vi "setSerializedData.vi"(0 "reference":refnum<class "NoteNode.lvclass">, 1 "parent":refnum<class "AbstractNode.lvclass">, 2 "children":refnum<class "AbstractNode.lvclass">[](array[class]), 3 "xmlOut":string, 5 "error in (no error)":errorcluster) -> (14 "reference out":refnum<class "NoteNode.lvclass">, 19 "error out":errorcluster)   [LabVIEW 2020, in "NoteNode.lvclass"]
doc: "setSerializedData"
uses:
  <resource>/Framework/Providers/Open_GDS/UML/NoteNode_class/NoteNode.lvclass
  C:/Program Files (x86)/National Instruments/LabVIEW 2020/resource/Framework/Providers/Open_GDS/UML/RectangularNode_class/RectangularNode.lvclass
  C:/Program Files (x86)/National Instruments/LabVIEW 2020/resource/Framework/Providers/Open_GDS/UML/AbstractNode_class/AbstractNode.lvclass
  <resource>/Framework/Providers/Open_GDS/UML/AbstractNode_class/AbstractNode.lvclass
  <resource>/Framework/Providers/Open_GDS/UML/General/Rectangle/Rectangle Rectangle2D.ctl
  <resource>/Framework/Providers/Open_GDS/UML/MultiLineString_class/JustificationType.ctl
  <resource>/Framework/Providers/Open_GDS/UML/MultiLineString_class/MultiLineString.lvclass
  <resource>/Framework/Providers/Open_GDS/UML/RectangularNode_class/RectangularNode.lvclass
panel:
  in  "emptyPointNodes":refnum<class "AbstractNode.lvclass">[](array[class])
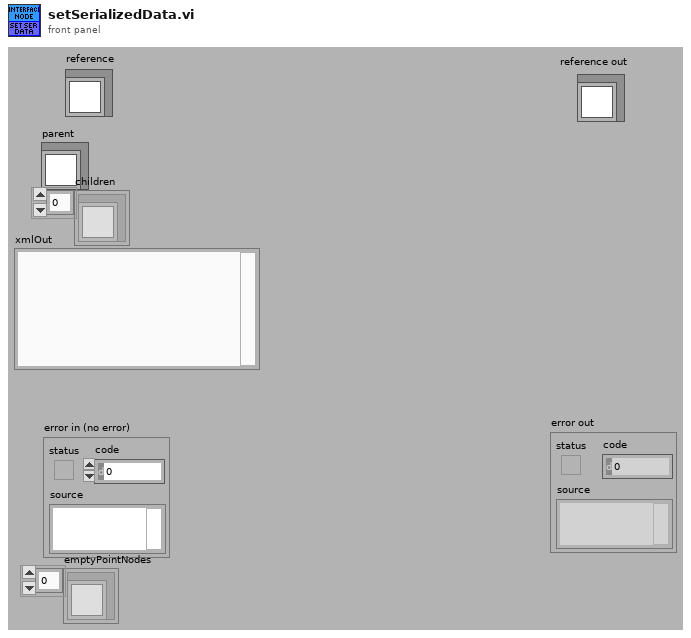
[diagram p1: front panel]
types:
  T1 = typedef "Rectangle Rectangle2D.ctl" = cluster{"x":dbl, "y":dbl, "width":dbl, "height":dbl}
  T2 = cluster{"Base class":cluster{"Base class":cluster{"parent":refnum<k1>, "children":refnum<k1>[], "Hidden":bool}, "bounds":T1}, "DEFAULT_WIDTH":i32, "DEFAULT_HEIGHT":i32, "DEFAULT_COLOR":u32, "FOLD_X":i32, "FOLD_Y":i32, "color":u32, "text":refnum<k1>, "pointNodes":refnum<k1>[]}
  T3 = typedef "MultiLineString.lvclass/JustificationType.ctl" = enum16{"LEFT", "CENTER", "RIGHT"}
  T4 = cluster{"Attributes":cluster{"Base class":cluster{"Base class":cluster{"parent":refnum<k1>, "children":refnum<k1>[], "Hidden":bool}, "bounds":T1}, "DEFAULT_WIDTH":i32, "DEFAULT_HEIGHT":i32, "DEFAULT_COLOR":u32, "FOLD_X":i32, "FOLD_Y":i32, "color":u32, "text":refnum<k1>, "pointNodes":refnum<k1>[]}, string}
  T5 = typedef "NoteNode.lvclass/ObjectAttributes.ctl" = cluster{"DEFAULT_WIDTH":i32, "DEFAULT_HEIGHT":i32, "DEFAULT_COLOR":u32, "FOLD_X":i32, "FOLD_Y":i32, "color":u32, "text":refnum<class "MultiLineString.lvclass">, "pointNodes":refnum<class "AbstractNode.lvclass">[]}
  T6 = typedef "RectangularNode.lvclass/ObjectAttributes.ctl" = cluster{"bounds":T1}
  T7 = typedef "AbstractNode.lvclass/ObjectAttributes.ctl" = cluster{"parent":refnum<class "AbstractNode.lvclass">, "children":refnum<class "AbstractNode.lvclass">[], "Hidden":bool}
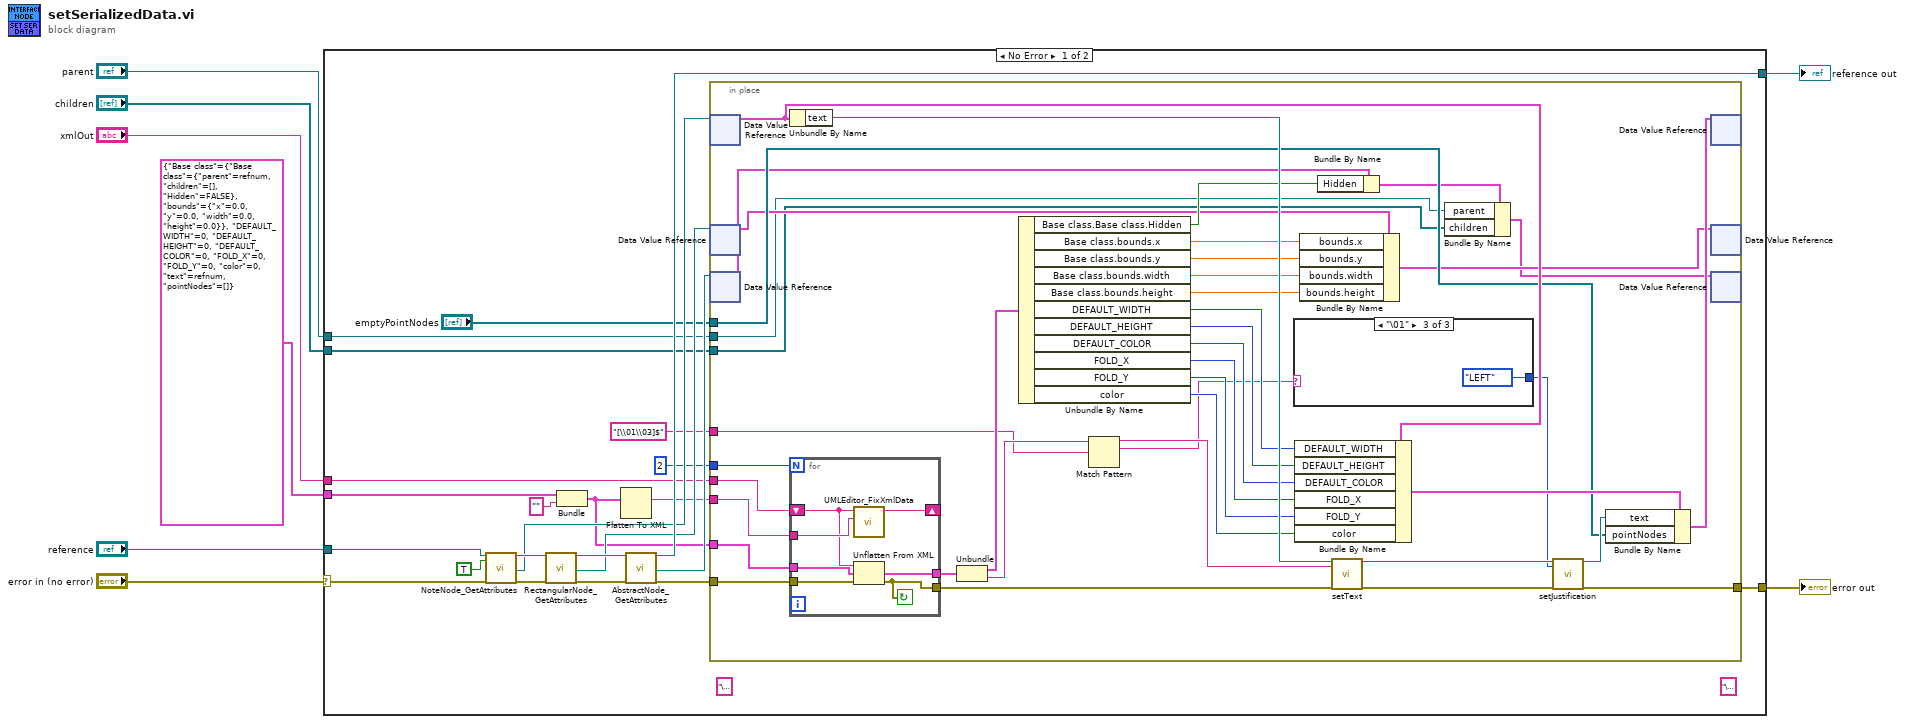
[diagram p0: block diagram]
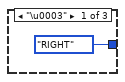
[diagram p2: hidden frame]
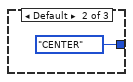
[diagram p3: hidden frame]
diagram:
  n1 = case shown="No Error" "error in (no error)" {
    selector: "error in (no error)" -> [w30 w82]
    tunnel: "reference" -> [w31 w83]
    tunnel: [w29 w82] -> w6
    tunnel: [w28 w83] -> w5
    tunnel: "xmlOut" -> [w11 _]
    tunnel: "parent" -> [w10 _]
    tunnel: "children" -> [w9 _]
    tunnel: T2 {"Base class"={"Base class"={"parent"=refnum, "children"=[], "Hidden"=FALSE}, "bounds"={"x"=0.0, "y"=0.0, "width"=0.0, "height"=0.0}}, "DEFAULT_WIDTH"=0, "DEFAULT_HEIGHT"=0, "DEFAULT_COLOR"=0, "FOLD_X"=0, "FOLD_Y"=0, "color"=0, "text"=refnum, "pointNodes"=[]} ("Attributes") -> [w26 _]
    frame No Error {
      (unwired) "\u0003"
      (unwired) "\u0001"
      n2 = call <resource>:"NoteNode_GetAttributes.vi"("reference in"=w31, "OnlyGetDvrReference(False)"=TRUE, "error in (no error)"=w30) -> ("reference out"=w24:refnum<class "NoteNode.lvclass">, "DataRef"=w20:refnum<data-value>, "error out"=w23:errorcluster)  [unwired: 13 in, 1 out]
      n3 = call <resource>:"RectangularNode_GetAttributes.vi"("reference in"=w24, "error in (no error)"=w23) -> ("reference out"=w22:refnum<class "NoteNode.lvclass">, "DataRef"=w19:refnum<data-value>, "error out"=w21:errorcluster)  [unwired: 14 in, 1 out]
      n4 = Bundle("Attributes"=w26, "") -> (w12:T4)  [unwired: 1 out]
      n5 = Flatten To XML(6:w12) -> (2:w13:string)
      n6 = call <resource>:"AbstractNode_GetAttributes.vi"("reference in"=w22, "error in (no error)"=w21) -> ("reference out"=w28:refnum<class "NoteNode.lvclass">, "DataRef"=w18:refnum<data-value>, "error out"=w14:errorcluster)  [unwired: 14 in, 1 out]
      n7 = in-place {
        in-place-border: "emptyPointNodes" -> [w57]
        in-place-border: "[\\01\\03]$" ("regular expression") -> [w48]
        in-place-border: 2 -> [w46]
        in-place-border: w14 -> [w45]
        in-place-border: w13 -> [w44]
        in-place-border: w12 -> [w43]
        in-place-border: w11 -> [w42]
        in-place-border: [w39] -> w29
        in-place-border: w10 -> [w35]
        in-place-border: w9 -> [w34]
        n8 = in-place-dvr #1(w20) -> (w71:T5)  [unwired: 1 out]
        n9 = in-place-dvr #2(w19) -> (w36:T6)  [unwired: 1 out]
        n10 = in-place-dvr #3(w18) -> (w38:T7)  [unwired: 1 out]
        n11 = Unbundle By Name(w71) -> ("text"=w70:refnum<class "MultiLineString.lvclass">)
        n12 = for {
          N: w46 -> [_]
          tunnel: w45 -> [w81]
          tunnel: [w77] -> w61
          tunnel: [w80] -> w41
          tunnel: w44 -> [w79]
          tunnel: w43 -> [w78]
          shift-right: [w76] -> _
          shift-left: w42 -> [w75]
          stop <- w77 continue-if-true
          n13 = call <resource>:"UMLEditor_FixXmlData.vi"("XmlTemplateIn"=w79, "xmlIn"=w75) -> ("XML OUt"=w76:string)  [unwired: 9 in]
          n14 = Unflatten From XML(xml string=w75, type=w78, error in (no error)=w81) -> (value=w80:T4, error out=w77:errorcluster)
        }
        n15 = Unbundle(w41) -> ("Attributes"=w55:T2, w49:string)
        n16 = Unbundle By Name(w55) -> ("Base class.Base class.Hidden"=w54:bool, "Base class.bounds.x"=w53:dbl, "Base class.bounds.y"=w52:dbl, "Base class.bounds.width"=w51:dbl, "Base class.bounds.height"=w50:dbl, "DEFAULT_WIDTH"=w69:i32, "DEFAULT_HEIGHT"=w68:i32, "DEFAULT_COLOR"=w67:u32, "FOLD_X"=w66:i32, "FOLD_Y"=w65:i32, "color"=w64:u32)
        n17 = Match Pattern(string=w49, regular expression=w48) -> (before substring=w62:string, match substring=w47:string)  [unwired: 3 out]
        n18 = case shown="\"\\01\"" w47 {
          tunnel: [JustificationType."RIGHT" ("justification") JustificationType."CENTER" ("justification") JustificationType."LEFT" ("justification")] -> w40
          frame "\u0003" {
          }
          frame Default {
          }
          frame "\u0001" {
          }
        }
        n19 = Bundle By Name(cluster=w71, "DEFAULT_WIDTH"=w69, "DEFAULT_HEIGHT"=w68, "DEFAULT_COLOR"=w67, "FOLD_X"=w66, "FOLD_Y"=w65, "color"=w64) -> (w63:T5)
        n20 = Bundle By Name(cluster=w36, "bounds.x"=w53, "bounds.y"=w52, "bounds.width"=w51, "bounds.height"=w50) -> (w33:T6)
        n21 = Bundle By Name(cluster=w38, "Hidden"=w54) -> (w37:T7)
        n22 = call-dynamic "setText.vi"("reference"=w70, "text"=w62, "error in (no error)"=w61) -> ("reference out"=w60:refnum<class "MultiLineString.lvclass">, "error out"=w59:errorcluster)  [unwired: 15 out]
        n23 = Bundle By Name(cluster=w37, "parent"=w35, "children"=w34) -> (w32:T7)
        n24 = call <resource>:"setJustification.vi"("reference"=w60, "justification"=w40, "error in (no error)"=w59) -> ("reference out"=w58:refnum<class "MultiLineString.lvclass">, "error out"=w39:errorcluster)  [unwired: 15 out]
        n25 = Bundle By Name(cluster=w63, "text"=w58, "pointNodes"=w57) -> (w56:T5)
        n26 = in-place-dvr #1(w56) -> ()  [unwired: 2 out]
        n27 = in-place-dvr #2(w33) -> ()  [unwired: 2 out]
        n28 = in-place-dvr #3(w32) -> ()  [unwired: 2 out]
      }
    }
    frame Error {
    }
  }
  "reference out" <- w5
  "error out" <- w6
